vi "Sollwerte aufbauen.vi"(8 "error in (no error)":errorcluster caption="Fehler (Eingang, kein Fehler)", 10 "Punkt":u8, 11 "Aktuelle Gasnummer":u8) -> (0 "error out":errorcluster caption="Fehler (Ausgang)")   [LabVIEW 2020, in "Linearisierung v2.lvlib" / "Gasteiler.lvlib" / "HovaCal.lvlib"]
uses:
  HovaCal.lvlib
  Aktion FGV Rohmesswerte sammeln.ctl
  HovaCAL_Interface/Kommunikation/Aktion FGV HovaCAL Interface Autolin.ctl
  HovaCAL_Interface/Kommunikation/Aktion_FGV_HovaCAL_Interface_GetData.ctl
  Linearisierung v2.lvlib
  Messdaten/Messdaten.lvlib
  Messdaten/Gewichtung (Stichprobe).ctl
  HovaCAL_Interface/Kommunikation/Kommunikation.lvlib
  HovaCAL_Interface/Helper/Helper.lvlib
  Gasteiler.lvlib
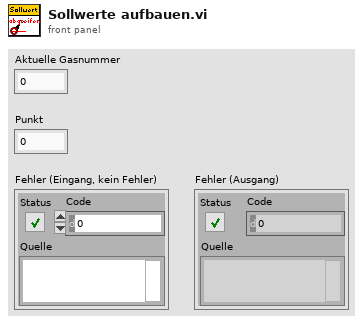
[diagram p1: front panel]
types:
  T1 = typedef "Linearisierung v2.lvlib/Gasteiler.lvlib/HovaCAL_Interface.lvlib/Kommunikation.lvlib/Aktion_FGV_HovaCAL_Interface_GetData.ctl" = enum16{"lesen", "SystemInfo", "MFC Info", "actual Values", "Limits", "first contact", "reset after read"}
  T2 = typedef "Linearisierung v2.lvlib/Gasteiler.lvlib/HovaCAL_Interface.lvlib/Kommunikation.lvlib/Aktion FGV HovaCAL Interface Autolin.ctl" = enum16{"lesen", "schreiben", "MFC Komponente fix setzen", "init"}
  T3 = typedef "Linearisierung v2.lvlib/Aktion FGV Rohmesswerte sammeln.ctl" = enum16{"lesen", "schreiben", "löschen", "Sollwert HovaCal"}
  T4 = typedef "Linearisierung v2.lvlib/Gasteiler.lvlib/HovaCAL_Interface.lvlib/Controls.lvlib/Info Cluster.ctl" = cluster{"device":string, "version":string, "number of mfc":i32, "number of pumps":i32, "number of temp controllers":i32, "number of mfs":i32, "number of balances":i32}
  T5 = typedef "Linearisierung v2.lvlib/KomponentenArray.ctl" = cluster{"Komponente:":T6, "Konzentration":dbl}[]
  T6 = typedef "Auswahlfeld.ctl" = u16
  T7 = typedef "Linearisierung v2.lvlib/HovaCAL Sollwerte je MFC Cluster.ctl" = cluster{"Sollwert je MFC1":sgl[], "Sollwert je MFC2":sgl[], "Sollwert je MFC3":sgl[], "Sollwert je MFC4":sgl[], "Sollwert je MFC5":sgl[], "Sollwert je Punpe1":sgl[], "Sollwert je Punpe2":sgl[]}
  T8 = typedef "Messdaten.lvlib/Gewichtung (Stichprobe).ctl" = enum16{"Sample", "Population"}
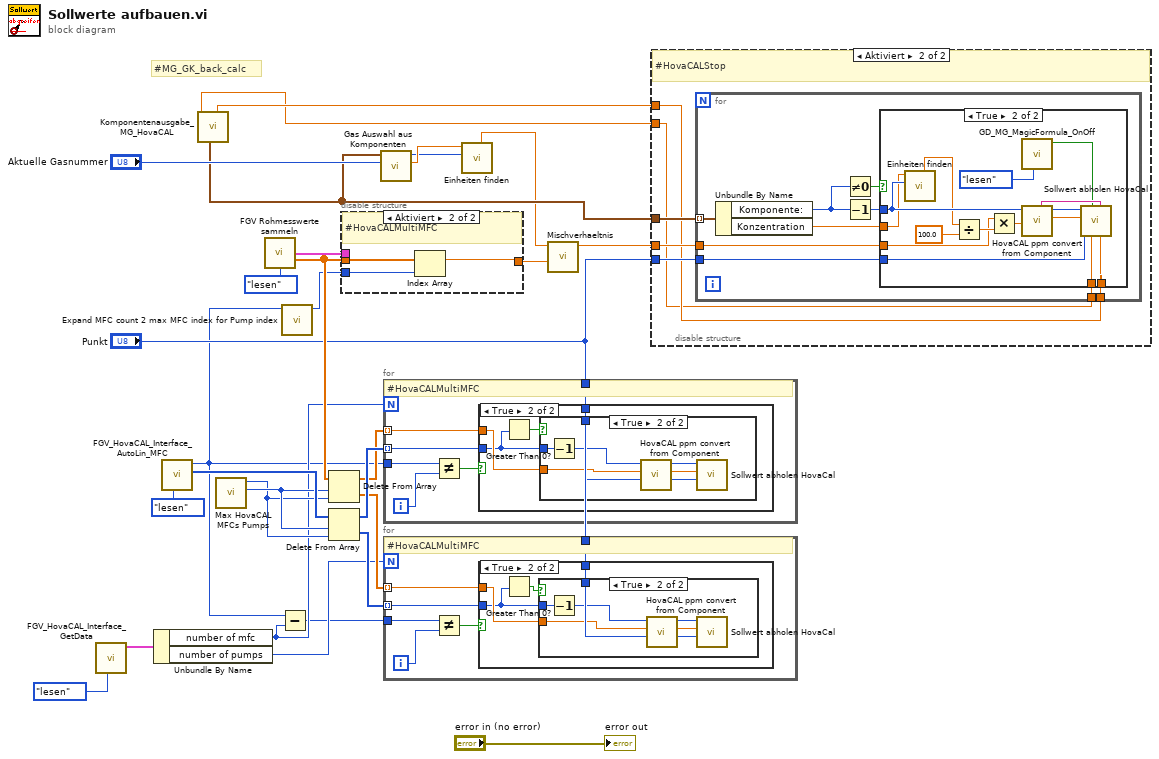
[diagram p0: block diagram]
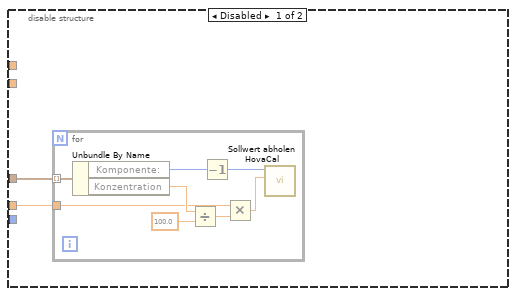
[diagram p6: hidden frame]
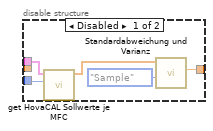
[diagram p8: hidden frame]
diagram:
  # "#MG_GK_back_calc"
  n1 = call "FGV_HovaCAL_Interface_GetData.vi"("Aktion"=Aktion_FGV_HovaCAL_Interface_GetData."lesen") -> ("System Cluster out"=w19:T4)  [unwired: 6 in, 4 out]
  n2 = Unbundle By Name(w19) -> ("number of mfc"=w11:i32, "number of pumps"=w13:i32)
  n3 = call "FGV_HovaCAL_Interface_AutoLin_MFC.vi"("Aktion"=Aktion_FGV_HovaCAL_Interface_Autolin."lesen") -> ("MFV Komponente fix out"=w23:u16[], "AutoLin MFC out"=w8:u16)  [unwired: 7 in, 2 out]
  n4 = call "Komponentenausgabe_MG_HovaCAL.vi"() -> ("höchste Konzentration Teilkomponente ppm"=w5:dbl, "Komponentenauswahl"=w6:T5, "GesamtKonzentration ppm"=w4:dbl)  [unwired: 3 in, 6 out]
  n5 = call "Max HovaCAL MFCs Pumps.vi"() -> ("max Pumps"=w15:i32, "max MFCs"=w14:i32)  [unwired: 10 in]
  n6 = call "FGV Rohmesswerte sammeln.vi"("Aktion"=Aktion_FGV_Rohmesswerte_sammeln."lesen") -> ("Sollwert je MFC Cluster"=w24:T7, "Aktueller Sollwert je MFC"=w18:dbl[])  [unwired: 11 in, 2 out]
  n7 = Subtract(x=w8, y=w11) -> (x-y=w10:i32)
  n8 = call "Expand MFC count 2 max MFC index for Pump index.vi"("AutoLin MFC"=w8) -> ("MFC idx"=w7:i32)  [unwired: 8 in, 2 out]
  n9 = Delete From Array(array=w18, length=w15, index=w14) -> (deleted portion=w16:dbl[], array with subset deleted=w17:dbl[])
  n10 = Delete From Array(array=w23, length=w15, index=w14) -> (deleted portion=w21:u16[], array with subset deleted=w22:u16[])
  n11 = disable-structure shown="Aktiviert" {
    disable-tunnel: [w33 w36] -> w28
    disable-tunnel: w18 -> [_ w37]
    disable-tunnel: w24 -> [w32 _]
    disable-tunnel: w7 -> [w31 w35]
    frame Disabled {
      n12 = call "get HovaCAL Sollwerte je MFC.vi"("MFC in"=w31, "Sollwert je MFC Cluster"=w32) -> ("Sollwert MFC"=w30:sgl[])  [unwired: 9 in]
      n13 = call "Standardabweichung und Varianz.vi"("Gewichtung (Stichprobe)"=Gewichtung_(Stichprobe)."Sample", "X"=w30) -> ("Mittelwert"=w33:sgl)  [unwired: 7 in, 2 out]
    }
    frame Enabled {
      # "#HovaCALMultiMFC"
      n14 = Index Array(array=w37, index=w35) -> (element=w36:dbl)
    }
  }
  n15 = call "Gas Auswahl aus Komponenten.vi"("Gasnummer:"="Aktuelle Gasnummer", "Komponentenauswahl"=w6) -> ("Konzentration"=w3:dbl, "Auswahl"=w2:T6)  [unwired: 7 in, 1 out]
  n16 = for {
    N: w11 -> [_]
    tunnel: w8 -> [w42]
    tunnel: w17 -> [w40] mode=indexing
    tunnel: "Punkt" -> [w39]
    tunnel: w22 -> [w38] mode=indexing
    i -> [w43]
    # "#HovaCALMultiMFC"
    n17 = Not Equal?(x=w42, y=w43) -> (x != y?=w41:bool)
    n18 = case shown="True" w41 {
      tunnel: w40 -> [_ w47]
      tunnel: w39 -> [_ w46]
      tunnel: w38 -> [_ w44]
      frame False {
      }
      frame True {
        n19 = Greater Than 0?(x=w44) -> (x > 0?=w45:bool)
        n20 = case shown="True" w45 {
          tunnel: w47 -> [_ w49]
          tunnel: w46 -> [_ w53]
          tunnel: w44 -> [_ w52]
          frame False {
          }
          frame True {
            n21 = Decrement(x=w52) -> (x-1=w51:u16)
            n22 = call "HovaCAL ppm convert from Component.vi"("Konzentration"=w49, "Gasnummer"=w51) -> ("Konzentration in %"=w48:dbl, "Gasnummer out"=w50:T6)  [unwired: 5 in, 3 out]
            n23 = call "Sollwert abholen HovaCal.vi"("Punkt"=w53, "Sollwert"=w48, "Gasindex"=w50) -> ()  [unwired: 8 in, 1 out]
          }
        }
      }
    }
  }
  n24 = for {
    N: w13 -> [_]
    tunnel: w10 -> [w58]
    tunnel: w16 -> [w56] mode=indexing
    tunnel: "Punkt" -> [w55]
    tunnel: w21 -> [w54] mode=indexing
    i -> [w59]
    # "#HovaCALMultiMFC"
    n25 = Not Equal?(x=w58, y=w59) -> (x != y?=w57:bool)
    n26 = case shown="True" w57 {
      tunnel: w56 -> [_ w63]
      tunnel: w55 -> [_ w62]
      tunnel: w54 -> [_ w60]
      frame False {
      }
      frame True {
        n27 = Greater Than 0?(x=w60) -> (x > 0?=w61:bool)
        n28 = case shown="True" w61 {
          tunnel: w63 -> [_ w64]
          tunnel: w62 -> [_ w69]
          tunnel: w60 -> [_ w68]
          frame False {
          }
          frame True {
            n29 = Decrement(x=w68) -> (x-1=w67:u16)
            n30 = call "HovaCAL ppm convert from Component.vi"("Konzentration"=w64, "Gasnummer"=w67) -> ("Konzentration in %"=w65:dbl, "Gasnummer out"=w66:T6)  [unwired: 5 in, 3 out]
            n31 = call "Sollwert abholen HovaCal.vi"("Punkt"=w69, "Sollwert"=w65, "Gasindex"=w66) -> ()  [unwired: 8 in, 1 out]
          }
        }
      }
    }
  }
  n32 = call "Einheiten finden.vi"("Komponente"=w2, "Wert"=w3) -> ("Wert ppm"=w1:dbl)  [unwired: 5 in, 4 out]
  n33 = call "Mischverhaeltnis.vi"("Konzentration"=w28, "Sollwert"=w1) -> ("%"=w27:dbl)  [unwired: 8 in, 1 out]
  n34 = disable-structure shown="Aktiviert" {
    disable-tunnel: w6 -> [w71 w84]
    disable-tunnel: w27 -> [w70 w83]
    disable-tunnel: "Punkt" -> [_ w82]
    disable-tunnel: w5 -> [_ w81]
    disable-tunnel: w4 -> [_ w80]
    frame Disabled {
      n35 = for {
        tunnel: w71 -> [w79] mode=indexing
        tunnel: w70 -> [w74]
        n36 = Unbundle By Name(w79) -> ("Komponente:"=w78:T6, "Konzentration"=w75:dbl)
        n37 = Divide(x=w75, y=sgl 100.0) -> (x/y=w76:dbl)
        n38 = Decrement(x=w78) -> (x-1=w72:T6)
        n39 = Multiply(x=w74, y=w76) -> (x*y=w73:dbl)
        n40 = call "Sollwert abholen HovaCal.vi"("Sollwert"=w73, "Gasindex"=w72) -> ()  [unwired: 9 in, 1 out]
      }
    }
    frame Enabled {
      # "#HovaCALStop"
      n41 = for {
        tunnel: w84 -> [w93] mode=indexing
        tunnel: w83 -> [w86]
        tunnel: w82 -> [w89]
        tunnel: w81 -> [w88]
        tunnel: w80 -> [w87]
        n42 = Unbundle By Name(w93) -> ("Komponente:"=w91:T6, "Konzentration"=w85:dbl)
        n43 = Not Equal To 0?(x=w91) -> (x != 0?=w90:bool)
        n44 = Decrement(x=w91) -> (x-1=w92:T6)
        n45 = case shown="True" w90 {
          tunnel: w92 -> [_ w98]
          tunnel: w89 -> [_ w108]
          tunnel: w88 -> [_ w104]
          tunnel: w87 -> [_ w103]
          tunnel: w86 -> [_ w101]
          tunnel: w85 -> [_ w97]
          frame False {
          }
          frame True {
            n46 = call "Einheiten finden.vi"("Komponente"=w98, "Wert"=w97) -> ("Wert ppm"=w96:dbl)  [unwired: 5 in, 4 out]
            n47 = Divide(x=w96, y=sgl 100.0) -> (x/y=w102:dbl)
            n48 = Multiply(x=w101, y=w102) -> (x*y=w99:dbl)
            n49 = call "GD_MG_MagicFormula_OnOff.vi"("Aktion"=enum16{"lesen", "schreiben", "init"}."lesen") -> ("MG_use_magic_formula"=w95:bool)  [unwired: 8 in, 1 out]
            n50 = call "HovaCAL ppm convert from Component.vi"("Konzentration"=w99, "Gasnummer"=w98) -> ("Konzentration in %"=w106:dbl, "Gasnummer out"=w107:T6, "Einheit in String"=w105:string)  [unwired: 5 in, 2 out]
            n51 = call "Sollwert abholen HovaCal.vi"("höchste Konzentration Teilkomponente"=w104, "Einheit in String"=w105, "Gesamtkonzentration"=w103, "DoIt"=w95, "Punkt"=w108, "Sollwert"=w106, "Gasindex"=w107) -> ()  [unwired: 4 in, 1 out]
          }
        }
      }
    }
  }
  "error out" <- "error in (no error)"
